vi "Finish.vi"(8 "error in (no error)":errorcluster, 11 "System in":refnum<class "System.lvclass">) -> (0 "error out":errorcluster, 3 "System out":refnum<class "System.lvclass">)   [LabVIEW 2013, in "System.lvlib" / "System.lvclass"]
uses:
  System.lvclass
  SystemStates.ctl
  System.lvclass/System.ctl
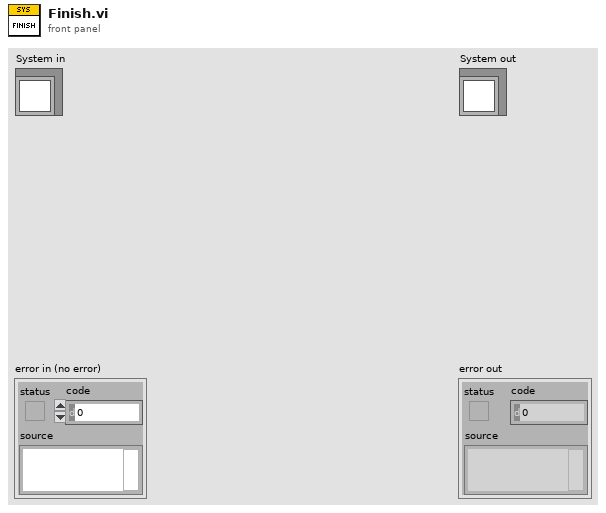
[diagram p1: front panel]
types:
  T1 = typedef "System.lvlib/System.lvclass/SystemStates.ctl" = enum16{"Unknown", "Running", "Stopped"}
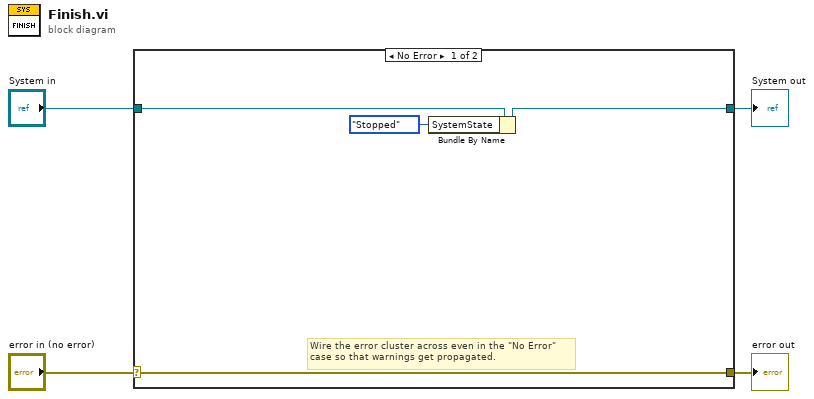
[diagram p0: block diagram]
diagram:
  n1 = case shown="No Error" "error in (no error)" {
    selector: "error in (no error)" -> [w7 w10]
    tunnel: [w7 w10] -> w3
    tunnel: [w6 w9] -> w1
    tunnel: "System in" -> [w8 w9]
    frame No Error {
      # "Wire the error cluster across even in the \"No Error\"\ncase so that warnings get propagated."
      n2 = Bundle By Name(cluster=w8, "SystemState"=SystemStates."Stopped") -> (w6:refnum<class "System.lvclass">)
    }
    frame Error {
    }
  }
  "error out" <- w3
  "System out" <- w1
